vi "Read UI references.vi"(8 "error in (no error)":errorcluster, 11 "PD-Data in":refnum<class "PD-Main.lvclass">) -> (0 "error out":errorcluster, 2 "UI references":T1, 3 "PD-Data out":refnum<class "PD-Main.lvclass">)   [LabVIEW 2013, in "PowderDeposition.lvlib" / "PD-Main.lvclass"]
uses:
  PD-Main.lvclass
  UI-references.ctl
  Assembly/Motor-selection.ctl
  Motor-status.ctl
  Action/Motor-actions.ctl
  Options.ctl
  PD-Main.lvclass/PD-Main.ctl
  Assembly/Motor-assembly.lvclass
  Action/Action.lvclass
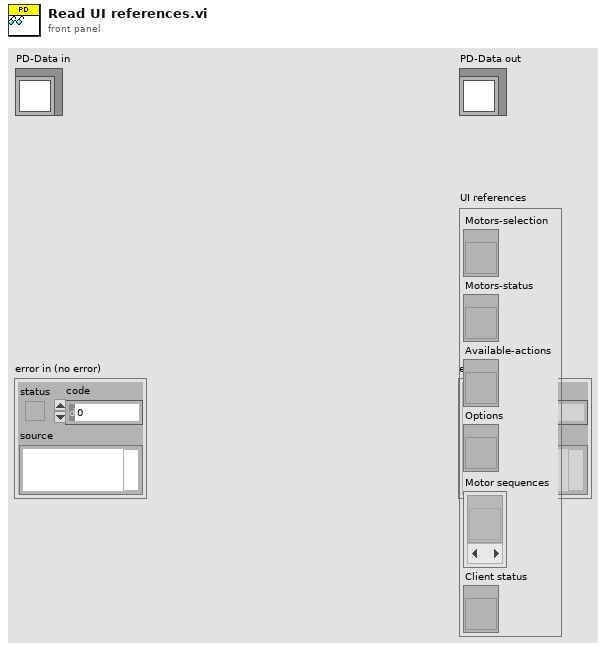
[diagram p1: front panel]
types:
  T1 = typedef "PowderDeposition.lvlib/PD-Main.lvclass/UI-references.ctl" = cluster{"Motors-selection":refnum<vi>, "Motors-status":refnum<vi>, "Available-actions":refnum<vi>, "Options":refnum<vi>, "Motor sequences":refnum<vi>[], "Client status":refnum<vi>}
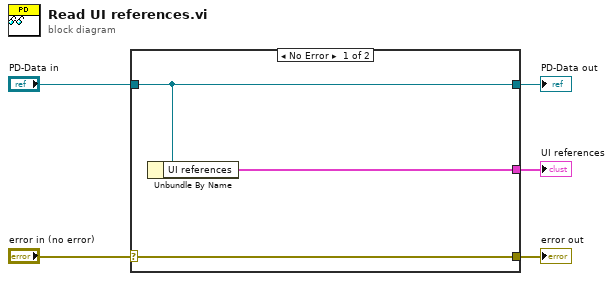
[diagram p0: block diagram]
diagram:
  n1 = case shown="No Error" "error in (no error)" {
    selector: "error in (no error)" -> [w8 w9]
    tunnel: [w8 w9] -> w4
    tunnel: [w7 w10] -> w2
    tunnel: "PD-Data in" -> [w7 w10]
    tunnel: [w6 _] -> w1
    frame No Error {
      n2 = Unbundle By Name(w7) -> ("UI references"=w6:T1)
    }
    frame Error {
    }
  }
  "error out" <- w4
  "PD-Data out" <- w2
  "UI references" <- w1
